vi "addString[]Element.vi"(7 "Name":string, 8 "error in (no error)":errorcluster, 9 "Value":string[](array[string]), 10 "Replace? (false)":bool, 11 "tBSONDocument in":refnum<class "tBSONDocument.lvclass">) -> (0 "error out":errorcluster, 3 "tBSONDocument out":refnum<class "tBSONDocument.lvclass">)   [LabVIEW 2013, in "BSON.lvlib" / "tBSONDocument.lvclass"]
doc: "Adds a string array to a BSON document."
uses:
  tBSONDocument.lvclass
  tBSONElement/tBSONElement.lvclass
  BSONElements/tBSONString/tBSONString.lvclass
  BSONElements/tBSONString/setValue.vi
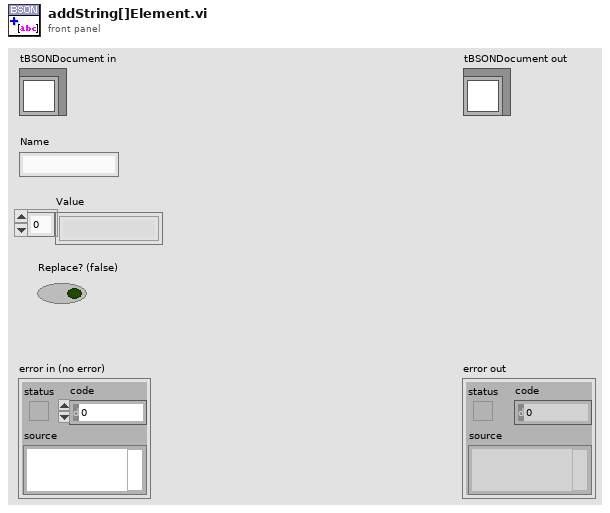
[diagram p1: front panel]
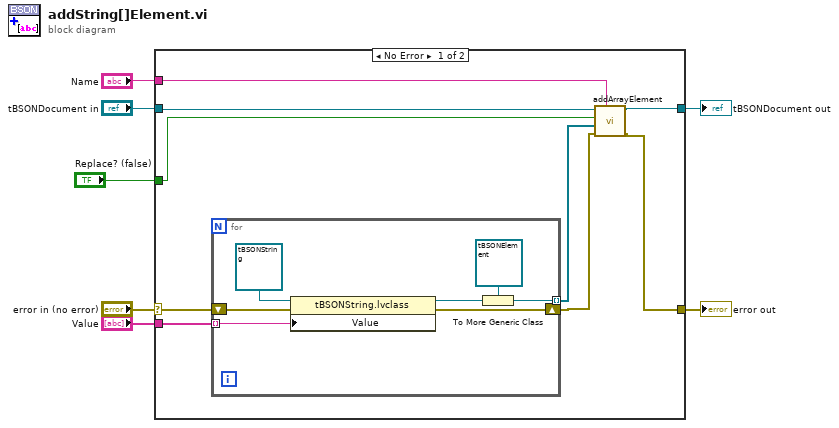
[diagram p0: block diagram]
diagram:
  n1 = case shown="No Error" "error in (no error)" {
    selector: "error in (no error)" -> [w15 w25]
    tunnel: [w11 w25] -> w6
    tunnel: [w10 w24] -> w4
    tunnel: "tBSONDocument in" -> [w14 w24]
    tunnel: "Value" -> [w16 _]
    tunnel: "Name" -> [w9 _]
    tunnel: "Replace? (false)" -> [w8 _]
    frame No Error {
      n2 = for {
        tunnel: w16 -> [w23] mode=indexing
        shift-right: [w21] -> w13
        shift-left: w15 -> [w22]
        tunnel: [w18] -> w12 mode=indexing
        n3 = property class="tBSONString.lvclass"(reference=refnum<class "tBSONString.lvclass"> refnum ("BSON.lvlib:tBSONString.lvclass"), error in=w22, "Value"=w23) -> (reference out=w20:refnum<class "tBSONString.lvclass">, error out=w21:errorcluster)
        n4 = To More Generic Class(target class=refnum<class "tBSONElement.lvclass"> refnum ("BSON.lvlib:tBSONElement.lvclass"), reference=w20) -> (generic class reference=w18:refnum<class "tBSONElement.lvclass">)
      }
      n5 = call "addArrayElement.vi"("Name"=w9, "error in (no error)"=w13, "Value"=w12, "Replace? (false)"=w8, "tBSONDocument in"=w14) -> ("error out"=w11:errorcluster, "tBSONDocument out"=w10:refnum<class "tBSONDocument.lvclass">)  [unwired: 5 in]
    }
    frame Error {
    }
  }
  "error out" <- w6
  "tBSONDocument out" <- w4
